vi "Update DataSeries Displayed in Plot.vi"(8 "error in":errorcluster, 9 "Tab Control":T3(ring), 10 "Plot Data":T1[][](array[typedef]), 11 "XYGraph Ref In":refnum<vi>) -> (0 "error out":errorcluster)   [LabVIEW 2017, in "DTacq Plot Display Library.lvlib"]
doc: "Updates the data that is displayed on the plot."
uses:
  DTacq Plot Display Library.lvlib
  Plot Data--Cluster.ctl
  Network Shared Variables/Typedefs/X and Y Variant Arrays--Cluster.ctl
  Network Shared Variables/Shared Variables Library.lvlib
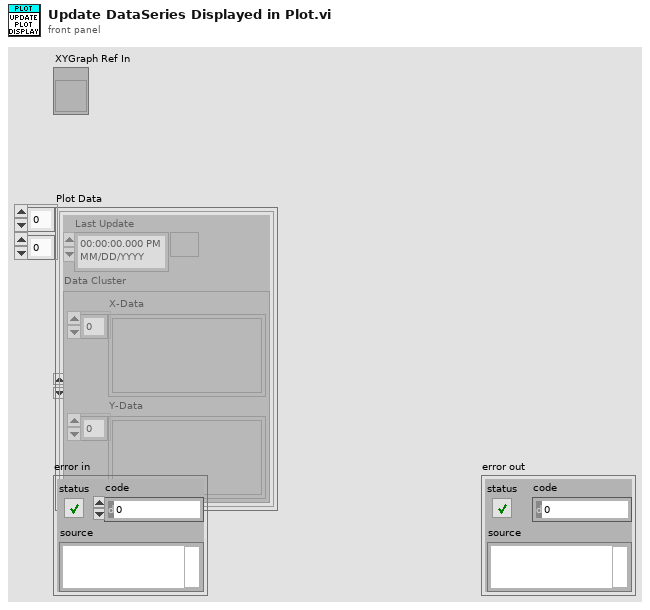
[diagram p1: front panel]
types:
  T1 = typedef "DTacq Plot Display Library.lvlib/Plot Data--Cluster.ctl" = cluster{"Last Update":timestamp, "Data Cluster":T2}
  T2 = typedef "Shared Variables Library.lvlib/X and Y Variant Arrays--Cluster.ctl" = cluster{"X-Data":variant[], "Y-Data":variant[]}
  T3 = enum32{"Page 1", "Page 2", "Page 3", "Page 4", "Page 5", "Page 6"}
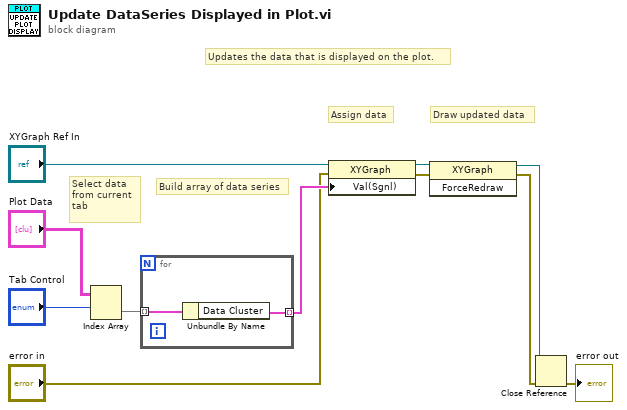
[diagram p0: block diagram]
diagram:
  # "Draw updated data"
  # "Assign data"
  # "Build array of data series"
  # "Select data\nfrom current\ntab"
  # "Updates the data that is displayed on the plot."
  n1 = Index Array(array="Plot Data", index (row)="Tab Control") -> (element=w11:T1[])  [unwired: 1 in]
  n2 = for {
    tunnel: w11 -> [w13] mode=indexing
    tunnel: [w12] -> w7 mode=indexing
    n3 = Unbundle By Name(w13) -> ("Data Cluster"=w12:T2)
  }
  n4 = property class="XYGraph"(reference="XYGraph Ref In", error in="error in", "Val(Sgnl)"=w7) -> (reference out=w6:refnum<vi>, error out=w5:errorcluster)
  n5 = invoke class="XYGraph" method="ForceRedraw"(reference=w6, error in=w5) -> (reference out=w3:refnum<vi>, error out=w2:errorcluster)  [unwired: 1 in, 1 out]
  n6 = Close Reference(reference=w3, error in (no error)=w2) -> (error out=→"error out":errorcluster)
